vi "Отладка ВП (Подпрограмма).vi"(1 "Число":dbl format="%.2f") -> (0 "Результат":dbl format="%.2f")   [LabVIEW 2017]
doc: "This VI is a subVI for an exercise in the LabVIEW Basics I course.\n\nThis exercise is used to demonstrate the use of different debugging tools. First, fix the broken run arrow and then use the different debugging tools to see how they work."
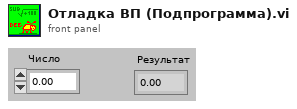
[diagram p1: front panel]
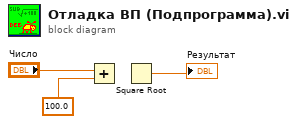
[diagram p0: block diagram]
diagram:
  n1 = Add(x="Число", y=100.0) -> ()  [unwired: 1 out]
  n2 = Square Root() -> (sqrt(x)=→"Результат":dbl)  [unwired: 1 in]
